vi "Digital - SW-Timed Output.vi"() -> ()   [LabVIEW 2014]
doc: "This example demonstrates how to generate digital output data using software timing.\n\nFor instructions on how to connect your signals from the DAQ device, refer to your device documentation."
uses:
  <vilib>/Utility/error.llb/DialogType.ctl
  <vilib>/DAQmx/create/channels.llb/DAQmx Create Channel (DO-Digital Output).vi
  <vilib>/DAQmx/write.llb/DAQmx Write (Digital 1D Bool 1Chan 1Samp).vi
panel:
  in  "Output Array":bool[](array[boolean])=[FALSE, FALSE, FALSE, FALSE, FALSE, FALSE, FALSE, FALSE]
  in  "Stop":bool
  in  "Line(s)":tag="Dev1/port0/line0:7"
  # "Channel Settings"
  # "Data to Write"
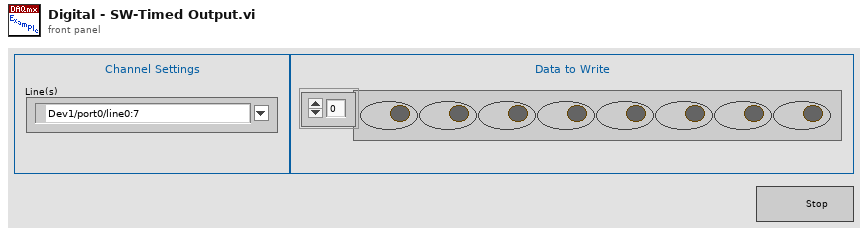
[diagram p1: front panel]
types:
  T1 = typedef "DialogType.ctl" = u16
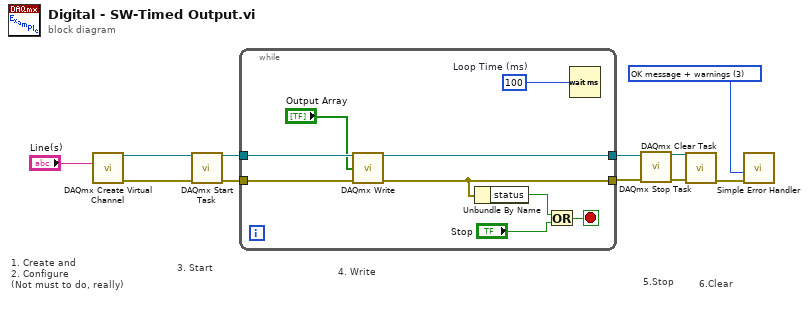
[diagram p0: block diagram]
diagram:
  w1 = T1 3 items=["no dialog", "OK message", "continue or stop message", "OK message + warnings", "continue/stop + warnings"] ("type of dialog (OK msg:1)")
  # "6.Clear"
  # "5.Stop"
  # "3. Start"
  # "4. Write"
  # "1. Create and \n2. Configure\n(Not must to do, really)"
  n1 = call-poly <vilib>:"DAQmx Create Virtual Channel.vi"("lines"="Line(s)") -> ("task out"=w6:refnum<k21>, "error out"=w7:errorcluster)  [unwired: 13 in]
  n2 = call <vilib>:"DAQmx Start Task.vi"("task/channels in"=w6, "error in"=w7) -> ("task out"=w11:refnum<k21>, "error out"=w10:errorcluster)  [unwired: 12 in]
  n3 = while {
    tunnel: w11 -> [w20]
    tunnel: w10 -> [w19]
    tunnel: [w16] -> w2
    tunnel: [w17] -> w3
    stop <- w18 stop-if-true
    w13 = u32 100  # Loop Time (ms)
    n4 = call-poly <vilib>:"DAQmx Write.vi"("task/channels in"=w20, "data"="Output Array", "error in"=w19) -> ("task out"=w17:refnum<k21>, "error out"=w16:errorcluster)  [unwired: 10 in, 1 out]
    n5 = Unbundle By Name(w16) -> ("status"=w15:bool)
    n6 = Or(x=w15, y="Stop") -> (x .or. y?=w18:bool)
    n7 = Wait (ms)(milliseconds to wait=w13) -> ()  [unwired: 1 out]
  }
  n8 = call <vilib>:"DAQmx Stop Task.vi"("task/channels in"=w3, "error in"=w2) -> ("task out"=w5:refnum<k21>, "error out"=w4:errorcluster)  [unwired: 12 in]
  n9 = call <vilib>:"DAQmx Clear Task.vi"("task in"=w5, "error in"=w4) -> ("error out"=w9:errorcluster)  [unwired: 13 in]
  n10 = call <vilib>:"Simple Error Handler.vi"("type of dialog (OK msg:1)"=w1, "error in (no error)"=w9) -> ()  [unwired: 3 in, 5 out]
